vi "HVenable.vi"(0 "Strings in":string[](array[string])=["C:\\CuspControl\\GPIB and Network\\Cusp\\HVpulser.txt", "6723"], 1 "Dubs in":dbl[](array[numeric])=[0.0, 10.0, 0.0]) -> ()   [LabVIEW 2018]
panel:
  in  "HVpulser file":path=path "C:/CuspControl/GPIB and Network/Cusp/HVpulser.txt"
  in  "Gain (15 V/V)":dbl=15.0
  out "Outvolts":dbl[](array[numeric])
  in  "Enable":bool
  in  "Amplitude (V)":dbl=10.0
  in  "Polarity":bool
  in  "subvi":bool=TRUE
  in  "ao lines":string[](array[string])=["ao0", "ao1", "ao2"]
  # "ao0\nao1\nao2"
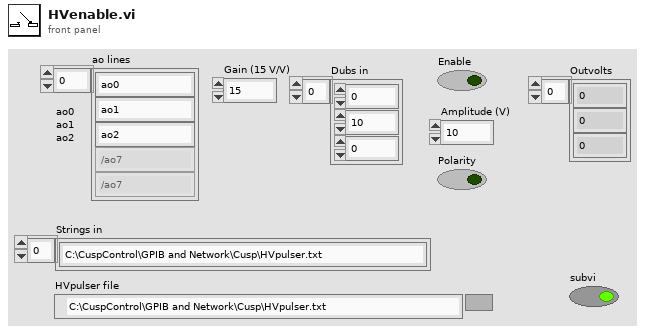
[diagram p1: front panel]
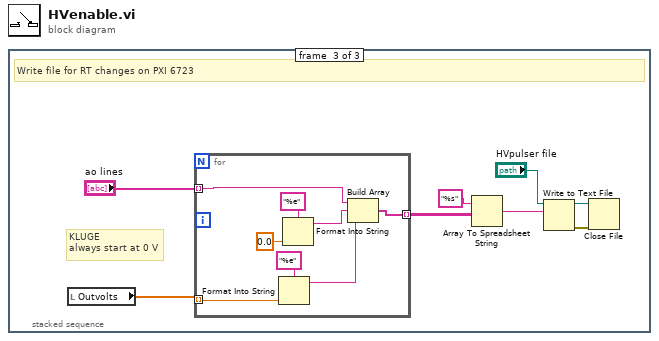
[diagram p0: block diagram]
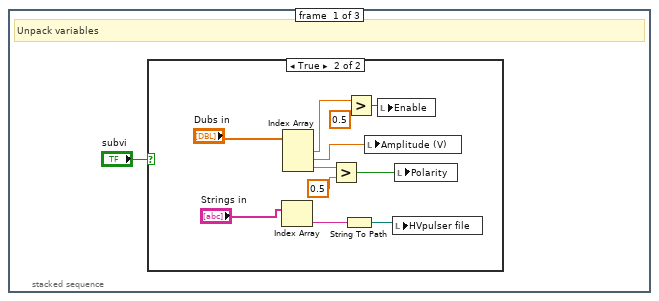
[diagram p2: hidden frame]
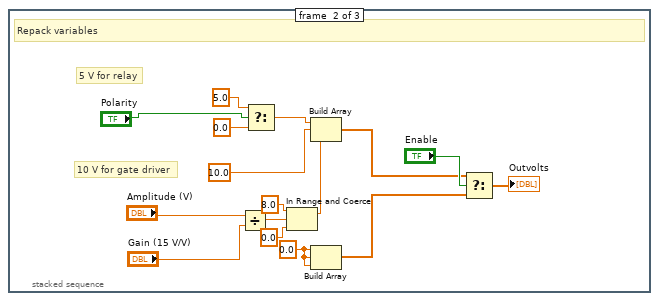
[diagram p4: hidden frame]
diagram:
  n1 = stacked-sequence {
    frame #0 {
      # "Unpack variables"
      n2 = case shown="True" "subvi" {
        frame False {
        }
        frame True {
          n3 = Index Array(array="Strings in") -> (element=w2:string)  [unwired: 1 in]
          n4 = Index Array(array="Dubs in") -> (element #1=w5:dbl, element #2=w4:dbl, element #3=w10:dbl)  [unwired: 3 in]
          n5 = Greater?(x=w10, y=0.5) -> (0:w8:bool)
          n6 = String To Path(string=w2) -> (path=w3:path)
          n7 = Greater?(x=w5, y=0.5) -> (0:w7:bool)
          n8 = local write "Amplitude (V)"(w4) -> ()
          n9 = local write "Enable"(w7) -> ()
          n10 = local write "HVpulser file"(w3) -> ()
          n11 = local write "Polarity"(w8) -> ()
        }
      }
    }
    frame #1 {
      w23 = 0.0 ("element")
      # "5 V for relay"
      # "10 V for gate driver"
      # "Repack variables"
      n12 = Divide(x="Amplitude (V)", y="Gain (15 V/V)") -> (x/y=w16:dbl)
      n13 = Select(t=5.0, s="Polarity", f=0.0) -> (s? t:f=w25:dbl)
      n14 = In Range and Coerce(upper limit=8.0, x=w16, lower limit=0.0) -> (coerced(x)=w15:dbl)  [unwired: 1 out]
      n15 = Build Array(w25, 10.0 ("t"), w15) -> (w21:dbl[])
      n16 = Build Array(w23, w23, w23) -> (w20:dbl[])
      n17 = Select(t=w21, s="Enable", f=w20) -> (s? t:f=→"Outvolts":dbl[])
    }
    frame #2 {
      # "KLUGE\nalways start at 0 V"
      # "Write file for RT changes on PXI 6723"
      n18 = local read "Outvolts"() -> (w35:dbl[])
      n19 = for {
        tunnel: "ao lines" -> [w43] mode=indexing
        tunnel: w35 -> [w40] mode=indexing
        tunnel: [w42] -> w29 mode=indexing
        n20 = Format Into String(format string="%e", w40) -> (resulting string=w38:string)  [unwired: 2 in, 1 out]
        n21 = Format Into String(format string="%e", 0.0 ("input 1")) -> (resulting string=w39:string)  [unwired: 2 in, 1 out]
        n22 = Build Array(w43, w39, w38) -> (w42:string[])
      }
      n23 = Array To Spreadsheet String(array=w29, 3:"%s" ("format string")) -> (spreadsheet string=w33:string)  [unwired: 1 in]
      n24 = Write to Text File(file (use dialog)="HVpulser file", text=w33) -> (refnum out=w32:refnum<file>, error out=w31:errorcluster)  [unwired: 2 in, 1 out]
      n25 = Close File(refnum=w32, error in=w31) -> ()  [unwired: 2 out]
    }
  }
